vi "NavX Query.vi"   [LabVIEW 2018]
uses:
  <vilib>/Rock Robotics/Network Tables/NT Read Boolean.vi
  <vilib>/Rock Robotics/Network Tables/NT Write Number.vi
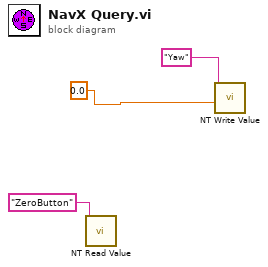
[diagram p0: block diagram]
diagram:
  n1 = call-poly <vilib>:"NT Read Value.vi"("Name"="ZeroButton") -> ()  [unwired: 9 in, 2 out]
  n2 = call-poly <vilib>:"NT Write Value.vi"("Numeric"=0.0, "Name"="Yaw") -> ()  [unwired: 9 in, 1 out]
